vi "Global ricalcola progressivo salvataggio.vi"() -> ()   [LabVIEW 2019]
panel:
  out "ricalcola progressivo durante salvataggio":bool
  # "variabile usata per ricalcolare il progressivo durante il salvataggio del collaudo\nin quanto potrebbe essere che nel banco 2, che ha 2 postazioni, durante il collaudo\nl'altra postazione salva un collaudo e quindi il progressivo calcolato prima del collaudo\nnon è più corretto."
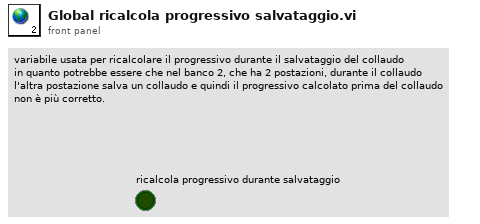
[diagram p1: front panel]
diagram:
